vi "AutoLin Messwerte FT-IR.vi"(10 "FT-IR Rohwerte":sgl[](array[numeric])) -> (2 "FT-IR Linearisiert":sgl[](array[numeric]))   [LabVIEW 2020, in "Linearisierung v2.lvlib"]
uses:
  Linearisierung v2.lvlib
  Aktionen Polynom Daten speichern.ctl
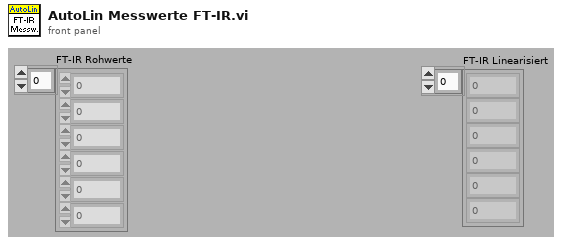
[diagram p1: front panel]
types:
  T1 = typedef "Linearisierung v2.lvlib/Aktionen Polynom Daten speichern.ctl" = enum16{"lesen", "laden", "speichern", "schreiben", "schreiben alle", "Liste erstellen", "aktivieren", "deaktivieren", "aktiv abfragen"}
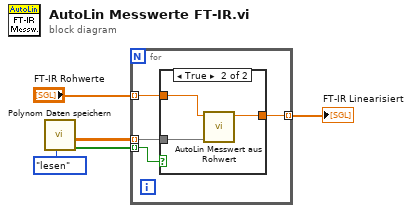
[diagram p0: block diagram]
diagram:
  n1 = call "Polynom Daten speichern.vi"("Aktionen"=Aktionen_Polynom_Daten_speichern."lesen") -> ("Aktiv"=w4:bool[], "Polynome"=w3:dbl[][])  [unwired: 5 in, 4 out]
  n2 = for {
    tunnel: "FT-IR Rohwerte" -> [w9] mode=indexing
    tunnel: w4 -> [w7] mode=indexing
    tunnel: w3 -> [w8] mode=indexing
    tunnel: [w6] -> w2 mode=indexing
    n3 = case shown="True" w7 {
      tunnel: w9 -> [w10 w13]
      tunnel: w8 -> [_ w12]
      tunnel: [w10 w11] -> w6
      frame False {
      }
      frame True {
        n4 = call "AutoLin Messwert aus Rohwert.vi"("Polynomkoeff."=w12, "Rohwert (ppm)"=w13) -> ("Messwert (ppm) linearisiert"=w11:dbl)  [unwired: 9 in]
      }
    }
  }
  "FT-IR Linearisiert" <- w2
